vi "Start SSR.vi"(0 "reference in":refnum<class "SSR.lvclass">, 5 "error in (no error)":errorcluster) -> (14 "reference out":refnum<class "SSR.lvclass">, 19 "error out":errorcluster)   [LabVIEW 2017, in "SSR.lvclass"]
uses:
  SSR.lvclass
  utils/SSR_Write.vi
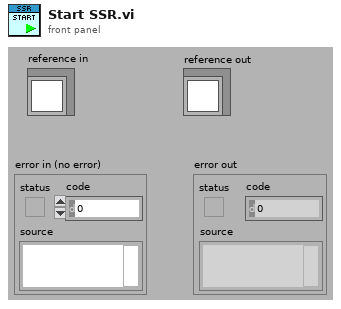
[diagram p1: front panel]
types:
  T1 = typedef "SSR.lvclass/ObjectAttributes.ctl" = cluster{"SSR Task":refnum<k21>, "SSR On/Off Status":bool, "Number of SSR Modules":u32, "Number of Total SSR Channels":u32, "SSR Module Names (NI-Max Name)":string[], "Number of Channels Per SSR Module":i32[], "SSR Status":bool[], "SSR Status to Set":bool[], "SSR VI Reference":refnum<vi>}
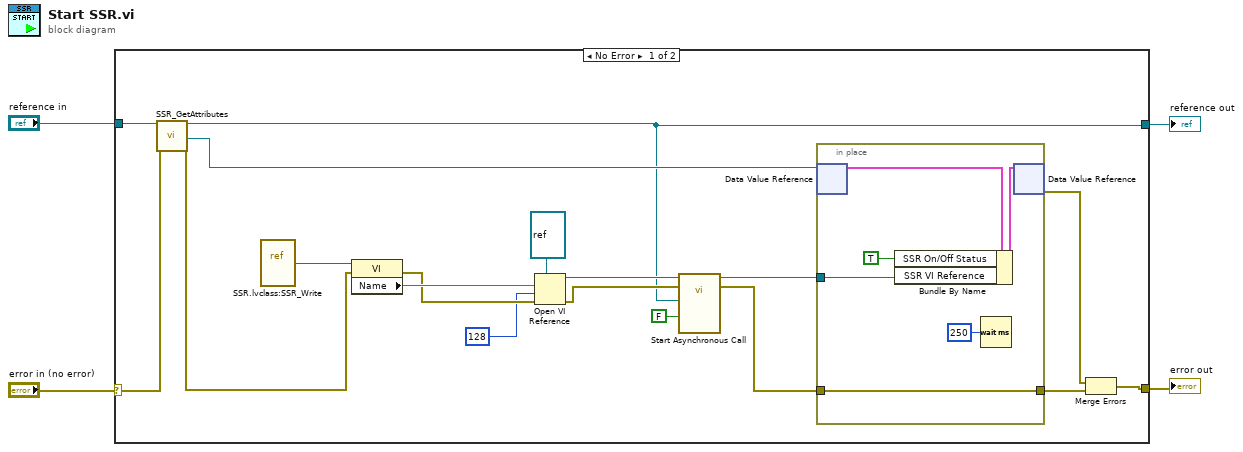
[diagram p0: block diagram]
diagram:
  n1 = case shown="No Error" "error in (no error)" {
    selector: "error in (no error)" -> [w21 w30]
    tunnel: [w19 w30] -> w3
    tunnel: [w6 w29] -> w1
    tunnel: "reference in" -> [w22 w29]
    frame No Error {
      n2 = call "SSR_GetAttributes.vi"("reference in"=w22, "error in (no error)"=w21) -> ("reference out"=w6:refnum<class "SSR.lvclass">, "DataRef"=w18:refnum<data-value>, "error out"=w11:errorcluster)  [unwired: 14 in, 1 out]
      n3 = vi-ref "SSR.lvclass:SSR_Write.vi"() -> (w14:refnum<vi>)
      n4 = property class="VI"(reference=w14, error in=w11) -> (error out=w13:errorcluster, "Name"=w15:string)  [unwired: 1 out]
      n5 = Open VI Reference(type specifier VI Refnum (for type only)=refnum<vi> refnum, vi path=w15, options=128, error in (no error)=w13) -> (vi reference=w9:refnum<vi>, error out=w7:errorcluster)  [unwired: 2 in]
      n6 = call-by-ref "Start Asynchronous Call"(reference=w9, error in=w7, "Stop SSR"=FALSE ("Stop Timer"), "reference in"=w6) -> (reference out=w5:refnum<vi>, error out=w10:errorcluster)  [unwired: 8 in, 2 out]
      n7 = in-place {
        in-place-border: w10 -> [w26]
        in-place-border: [w26] -> w17
        in-place-border: w5 -> [w24]
        n8 = in-place-dvr #1(w18) -> (w27:T1)  [unwired: 1 out]
        n9 = Bundle By Name(cluster=w27, "SSR On/Off Status"=TRUE, "SSR VI Reference"=w24) -> (w28:T1)
        n10 = Wait (ms)(milliseconds to wait=u32 250) -> ()  [unwired: 1 out]
        n11 = in-place-dvr #1(w28) -> (w20:errorcluster)  [unwired: 1 out]
      }
      n12 = Merge Errors(w20, w17) -> (w19:errorcluster)
    }
    frame Error {
    }
  }
  "error out" <- w3
  "reference out" <- w1
